vi "instr.DDS_FG.vi"(5 "SWITCH":string(combo), 7 "CH":enum16{"Channel A", "Channel B", "Both"}(ring), 8 "Error In":errorcluster caption="错误输入", 9 "FREQ":u32, 10 "AMP":u16, 11 "COM":refnum<visa-resource-name>) -> (0 "Error Out":errorcluster caption="错误输出", 3 "STA":bool)   [LabVIEW 2012, in "Lib_UEL.ATE.lvlib" / "Lib_Instrument.lvlib"]
uses:
  Lib_Instrument.lvlib
  <vilib>/Instr/_visa.llb/VISA Configure Serial Port (Instr).vi
panel:
  out "命令数":u8
  out "CMD":string[](array[string])
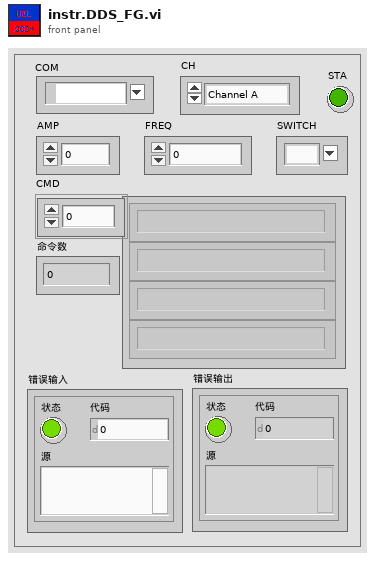
[diagram p1: front panel]
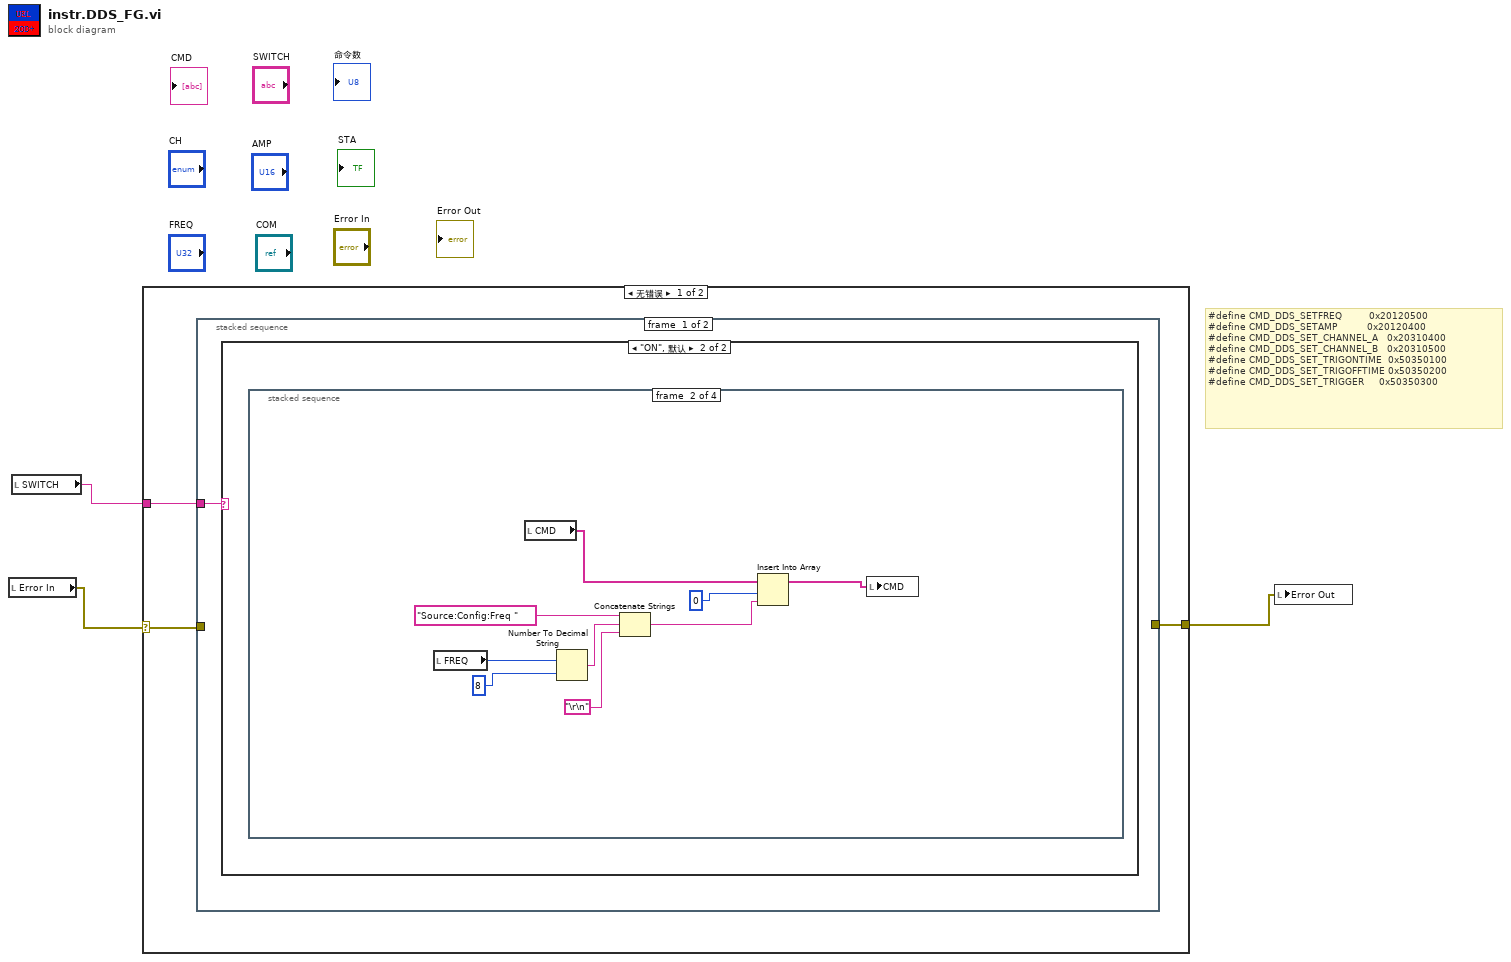
[diagram p0: block diagram]
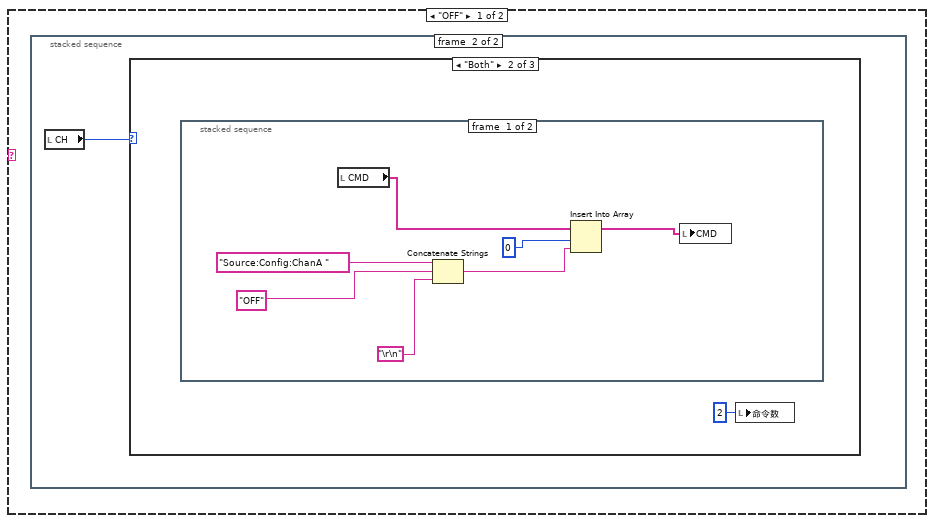
[diagram p2: hidden frame]
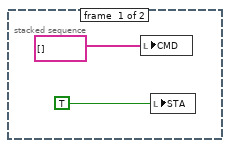
[diagram p3: hidden frame]
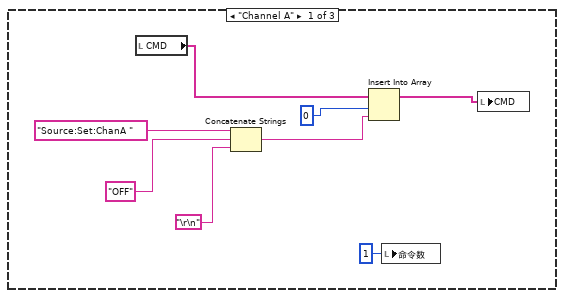
[diagram p4: hidden frame]
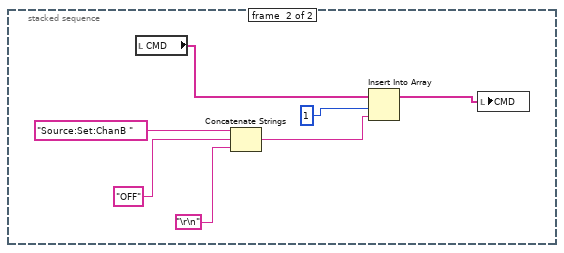
[diagram p5: hidden frame]
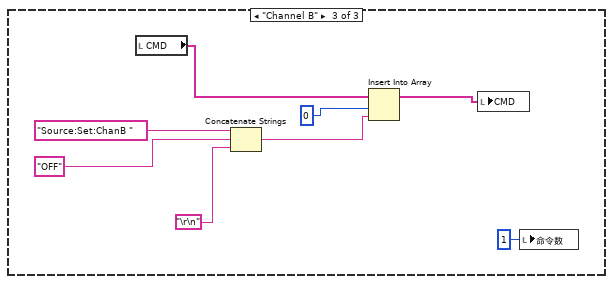
[diagram p6: hidden frame]
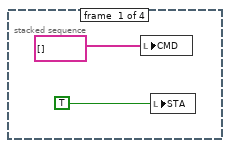
[diagram p7: hidden frame]
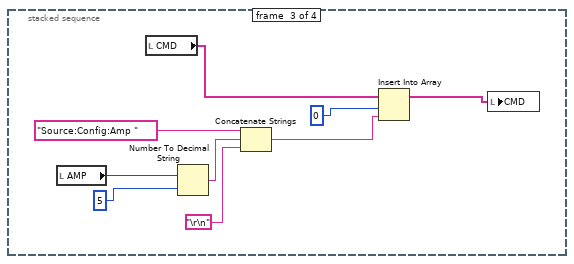
[diagram p8: hidden frame]
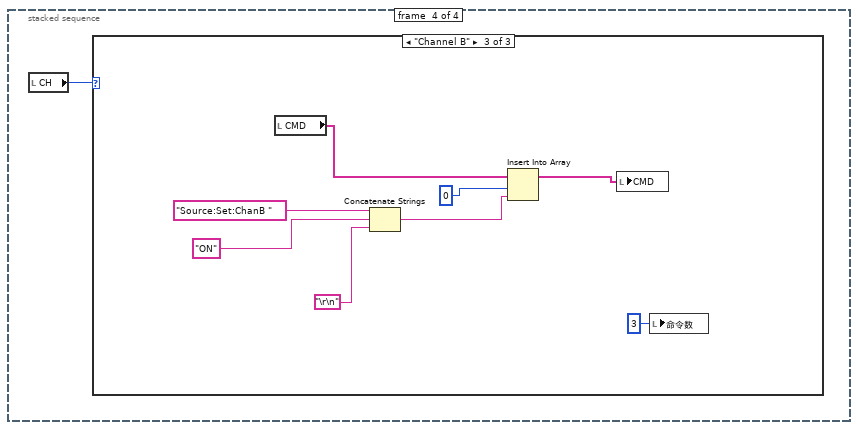
[diagram p9: hidden frame]
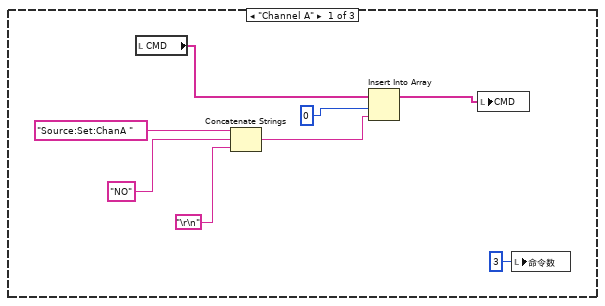
[diagram p10: hidden frame]
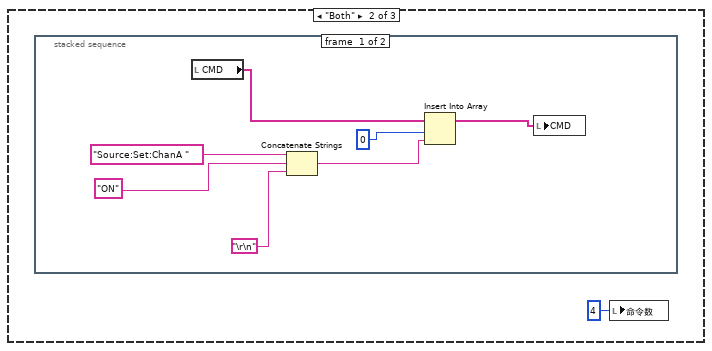
[diagram p11: hidden frame]
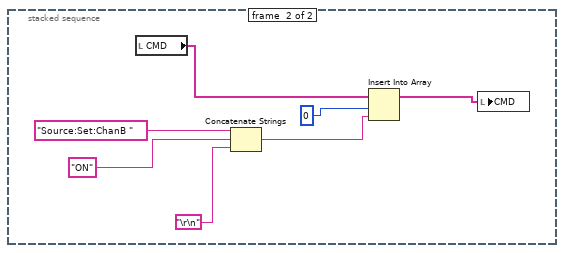
[diagram p12: hidden frame]
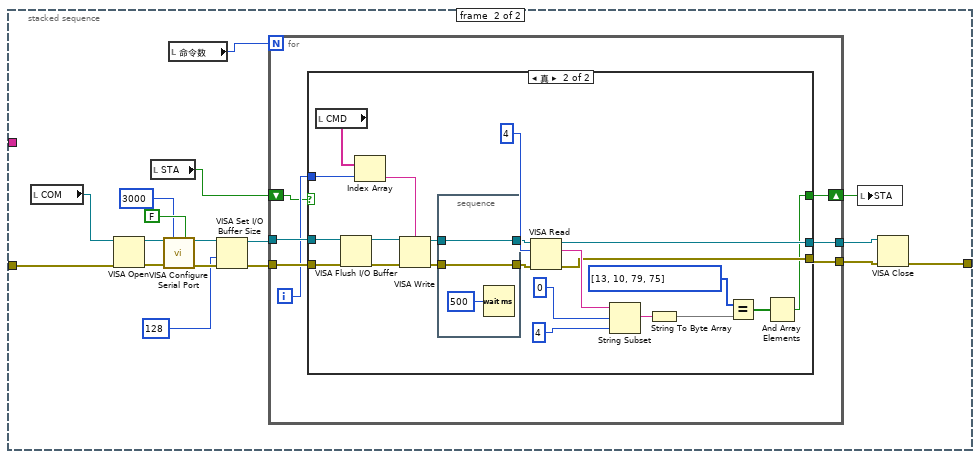
[diagram p13: hidden frame]
diagram:
  # "#define CMD_DDS_SETFREQ         0x20120500\n#define CMD_DDS_SETAMP          0x20120400\n#define CMD_DDS_SET_CHANNEL_A   0x20310400\n#define CMD_DDS_SET_CHANNEL_B   0x20310500\n#define CMD_DDS_SET_TRIGONTIME  0x50350100\n#define CMD_DDS_SET_TRIGOFFTIME 0x50350200\n#define CMD_DDS_SET_TRIGGER     0x50350300"
  n1 = local read "Error In"() -> (w2:errorcluster)
  n2 = local read "SWITCH"() -> (w3:string)
  n3 = case shown="无错误" w2 {
    selector: w2 -> [w6 w145]
    tunnel: w3 -> [w5 _]
    tunnel: [w4 w145] -> w1
    frame No Error {
      n4 = stacked-sequence {
        tunnel: w6 -> [_ w107]
        tunnel: w5 -> [w7 _]
        tunnel: [_ w103] -> w4
        frame #0 {
          n5 = case shown="\"ON\", 默认" w7 {
            frame "OFF" {
              n6 = stacked-sequence {
                frame #0 {
                  n7 = local write "CMD"(string[] []) -> ()
                  n8 = local write "STA"(TRUE ("STA")) -> ()
                }
                frame #1 {
                  n9 = local read "CH"() -> (w10:enum16{"Channel A", "Channel B", "Both"})
                  n10 = case shown="\"Both\"" w10 {
                    frame "Channel A" {
                      n11 = local read "CMD"() -> (w16:string[])
                      n12 = Concatenate Strings("Source:Set:ChanA " ("字符串"), "OFF" ("字符串"), "\r\n") -> (w15:string)
                      n13 = Insert Into Array(array=w16, index=0 ("索引"), new element=w15) -> (w13:string[])
                      n14 = local write "命令数"(u8 1 ("命令数")) -> ()
                      n15 = local write "CMD"(w13) -> ()
                    }
                    frame "Both" {
                      n16 = stacked-sequence {
                        frame #0 {
                          n17 = local read "CMD"() -> (w24:string[])
                          n18 = Concatenate Strings("Source:Config:ChanA " ("字符串"), "OFF" ("字符串"), "\r\n") -> (w23:string)
                          n19 = Insert Into Array(array=w24, index=0 ("索引"), new element=w23) -> (w21:string[])
                          n20 = local write "CMD"(w21) -> ()
                        }
                        frame #1 {
                          n21 = local read "CMD"() -> (w31:string[])
                          n22 = Concatenate Strings("Source:Set:ChanB " ("字符串"), "OFF" ("字符串"), "\r\n") -> (w30:string)
                          n23 = Insert Into Array(array=w31, index=1 ("索引"), new element=w30) -> (w28:string[])
                          n24 = local write "CMD"(w28) -> ()
                        }
                      }
                      n25 = local write "命令数"(u8 2 ("命令数")) -> ()
                    }
                    frame "Channel B" {
                      n26 = local read "CMD"() -> (w39:string[])
                      n27 = Concatenate Strings("Source:Set:ChanB " ("字符串"), "OFF" ("字符串"), "\r\n") -> (w38:string)
                      n28 = Insert Into Array(array=w39, index=0 ("索引"), new element=w38) -> (w36:string[])
                      n29 = local write "CMD"(w36) -> ()
                      n30 = local write "命令数"(u8 1 ("命令数")) -> ()
                    }
                  }
                }
              }
            }
            frame "ON", Default {
              n31 = stacked-sequence {
                frame #0 {
                  n32 = local write "CMD"(string[] []) -> ()
                  n33 = local write "STA"(TRUE ("STA")) -> ()
                }
                frame #1 {
                  n34 = local read "FREQ"() -> (w52:u32)
                  n35 = local read "CMD"() -> (w47:string[])
                  n36 = Number To Decimal String(number=w52, width (-)=i16 8 ("宽度(-)")) -> (decimal integer string=w49:string)
                  n37 = Concatenate Strings("Source:Config:Freq " ("字符串"), w49, "\r\n") -> (w46:string)
                  n38 = Insert Into Array(array=w47, index=0 ("索引"), new element=w46) -> (w44:string[])
                  n39 = local write "CMD"(w44) -> ()
                }
                frame #2 {
                  n40 = local read "AMP"() -> (w61:u16)
                  n41 = local read "CMD"() -> (w56:string[])
                  n42 = Number To Decimal String(number=w61, width (-)=i16 5 ("宽度(-)")) -> (decimal integer string=w58:string)
                  n43 = Concatenate Strings("Source:Config:Amp " ("字符串"), w58, "\r\n") -> (w55:string)
                  n44 = Insert Into Array(array=w56, index=0 ("索引"), new element=w55) -> (w53:string[])
                  n45 = local write "CMD"(w53) -> ()
                }
                frame #3 {
                  n46 = local read "CH"() -> (w62:enum16{"Channel A", "Channel B", "Both"})
                  n47 = case shown="\"Channel B\"" w62 {
                    frame "Channel A" {
                      n48 = local read "CMD"() -> (w68:string[])
                      n49 = Concatenate Strings("Source:Set:ChanA " ("字符串"), "NO" ("字符串"), "\r\n") -> (w67:string)
                      n50 = Insert Into Array(array=w68, index=0 ("索引"), new element=w67) -> (w65:string[])
                      n51 = local write "CMD"(w65) -> ()
                      n52 = local write "命令数"(u8 3 ("命令数")) -> ()
                    }
                    frame "Both" {
                      n53 = stacked-sequence {
                        frame #0 {
                          n54 = local read "CMD"() -> (w76:string[])
                          n55 = Concatenate Strings("Source:Set:ChanA " ("字符串"), "ON", "\r\n") -> (w75:string)
                          n56 = Insert Into Array(array=w76, index=0 ("索引"), new element=w75) -> (w73:string[])
                          n57 = local write "CMD"(w73) -> ()
                        }
                        frame #1 {
                          n58 = local read "CMD"() -> (w83:string[])
                          n59 = Concatenate Strings("Source:Set:ChanB " ("字符串"), "ON", "\r\n") -> (w82:string)
                          n60 = Insert Into Array(array=w83, index=0 ("索引"), new element=w82) -> (w80:string[])
                          n61 = local write "CMD"(w80) -> ()
                        }
                      }
                      n62 = local write "命令数"(u8 4 ("命令数")) -> ()
                    }
                    frame "Channel B" {
                      n63 = local read "CMD"() -> (w91:string[])
                      n64 = Concatenate Strings("Source:Set:ChanB " ("字符串"), "ON", "\r\n") -> (w90:string)
                      n65 = Insert Into Array(array=w91, index=0 ("索引"), new element=w90) -> (w88:string[])
                      n66 = local write "CMD"(w88) -> ()
                      n67 = local write "命令数"(u8 3 ("命令数")) -> ()
                    }
                  }
                }
              }
            }
          }
        }
        frame #1 {
          n68 = local read "COM"() -> (w108:refnum<visa-resource-name>)
          n69 = VISA Open(error in (no error)=w107, VISA resource name=w108) -> (VISA resource name=w110:refnum<visa-resource-name>, error out=w109:errorcluster)  [unwired: 3 in]
          n70 = local read "STA"() -> (w106:bool)
          n71 = call-poly "VISA Configure Serial Port"("VISA resource name"=w110, "timeout (10sec)"=u32 3000, "Enable Termination\nChar (T)"=FALSE ("Enable Termination\nChar (T)"), "error in (no error)"=w109) -> ("VISA resource name out"=w99:refnum<visa-resource-name>, "error out"=w100:errorcluster)  [unwired: 10 in]
          n72 = local read "命令数"() -> (w95:u8)
          n73 = VISA Set I/O Buffer Size(VISA resource name=w99, size (4096)=u32 128 ("大小(4096)"), error in (no error)=w100) -> (VISA resource name out=w98:refnum<visa-resource-name>, error out=w97:errorcluster)  [unwired: 1 in]
          n74 = for {
            N: w95 -> [_]
            tunnel: w97 -> [w117]
            tunnel: w98 -> [w116]
            shift-right: [w113] -> w102
            shift-left: w106 -> [w114]
            tunnel: [w112] -> w105
            tunnel: [w111] -> w104
            i -> [w115]
            n75 = case shown="真" w114 {
              selector: w114 -> [w120 _]
              tunnel: w117 -> [w118 w141]
              tunnel: w116 -> [w119 w131]
              tunnel: w115 -> [_ w140]
              tunnel: [w120 w122] -> w113
              tunnel: [w119 w134] -> w112
              tunnel: [w118 w133] -> w111
              frame False {
              }
              frame True {
                n76 = local read "CMD"() -> (w138:string[])
                n77 = VISA Flush I/O Buffer(VISA resource name=w131) -> (VISA resource name out=w130:refnum<visa-resource-name>)  [unwired: 2 in, 1 out]
                n78 = Index Array(array=w138, index=w140) -> (element=w139:string)
                n79 = VISA Write(VISA resource name=w130, write buffer=w139, error in (no error)=w141) -> (VISA resource name out=w128:refnum<visa-resource-name>, error out=w126:errorcluster)  [unwired: 1 out]
                n80 = stacked-sequence {
                  tunnel: [w144] -> w129
                  tunnel: w128 -> [w144]
                  tunnel: [w143] -> w127
                  tunnel: w126 -> [w143]
                  frame #0 {
                    n81 = Wait (ms)(milliseconds to wait=u32 500 ("等待时间（毫秒）")) -> ()  [unwired: 1 out]
                  }
                }
                n82 = VISA Read(VISA resource name=w129, byte count=u32 4 ("字节总数"), error in (no error)=w127) -> (VISA resource name out=w134:refnum<visa-resource-name>, read buffer=w137:string, error out=w133:errorcluster)  [unwired: 1 out]
                n83 = String Subset(string=w137, offset (0)=0 ("偏移量(0)"), length (rest)=4 ("长度（剩余）")) -> (substring=w124:string)
                n84 = String To Byte Array(string=w124) -> (unsigned byte array=w125:u8[])
                n85 = Equal?(x=u8[] [13, 10, 79, 75], y=w125) -> (x = y?=w123:bool[])
                n86 = And Array Elements(Boolean array=w123) -> (logical AND=w122:bool)
              }
            }
          }
          n87 = local write "STA"(w102) -> ()
          n88 = VISA Close(VISA resource name=w105, error in (no error)=w104) -> (error out=w103:errorcluster)
        }
      }
    }
    frame Error {
    }
  }
  n89 = local write "Error Out"(w1) -> ()
